vi "send_health_AURA.vi"(0 "TEMPERATURA":bool, 1 "Parametros AuraWheel":string[](array[string])=["nem1234", "test_rest", "http://api.aurawheel.dev/services/devices/status"], 2 "all rows":dbl[][](array[numeric]), 3 "WHEEL_SENSOR":bool, 4 "LIMITE MAX":dbl, 5 "LIMITE MIN":dbl, 6 "RFID_Error":errorcluster, 7 "FOTOCELULA":bool, 8 "RFID_LR6_Error":errorcluster, 9 "ESCRITURA ERROR":errorcluster, 10 "FPGA ERROR":errorcluster) -> (14 "JSON String Out":string, 15 "Response headers":string, 16 "error AURA":errorcluster)   [LabVIEW 2015]
uses:
  AURA_Wheel/Json2Labv.lvlib
panel:
  in  "DC":bool
  out "data":cluster{"status":string}
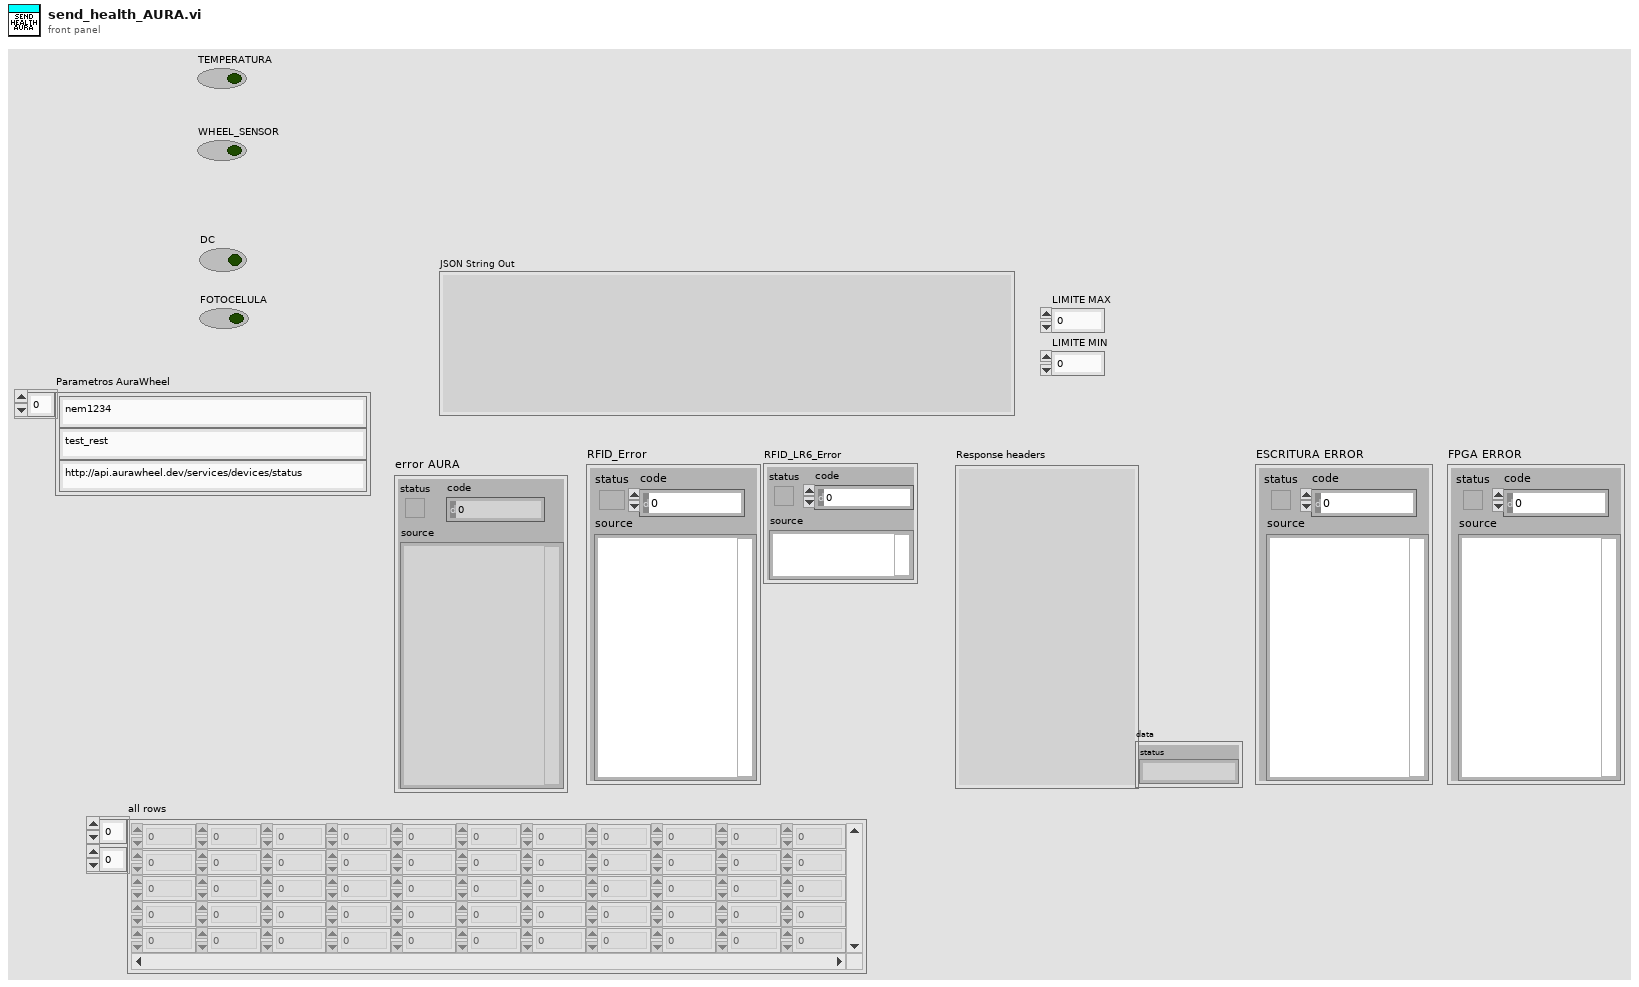
[diagram p1: front panel]
types:
  T1 = cluster{"g_st":dbl, "g_ts":dbl, "ds_id":string, "ds_st":dbl, "ds_ts":dbl, "ds_ss":cluster{"ss_tp":string, "ss_st":dbl, "ss_sl":string}[]}
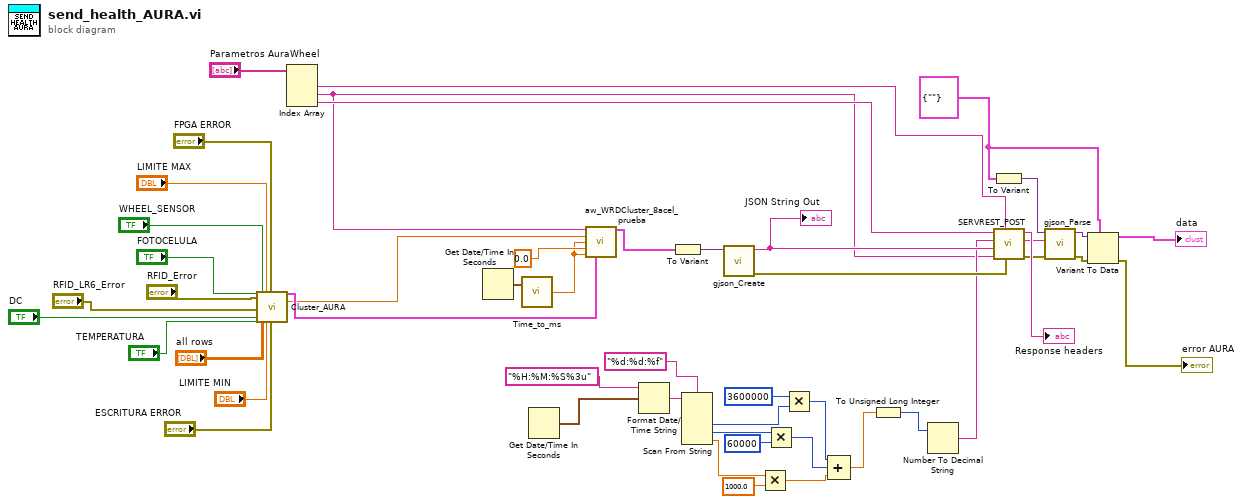
[diagram p0: block diagram]
diagram:
  w21 = cluster{"status":string} {"status"=""}
  n1 = call "Cluster_AURA.vi"("FOTOCELULA"="FOTOCELULA", "RFID_Error"="RFID_Error", "RFID_LR6_Error"="RFID_LR6_Error", "DC"="DC", "TEMPERATURA"="TEMPERATURA", "WHEEL_SENSOR"="WHEEL_SENSOR", "all rows"="all rows", "LIMITE MAX"="LIMITE MAX", "LIMITE MIN"="LIMITE MIN", "ERROR FPGA"="FPGA ERROR", "ERROR ESCRITURA"="ESCRITURA ERROR") -> ("appended array"=w45:cluster{string, dbl, "output string":string}[], "ESTADO WRD"=w11:dbl)  [unwired: 15 in]
  n2 = Index Array(array="Parametros AuraWheel") -> (element #1=w39:string, element #2=w4:string, element #3=w6:string)  [unwired: 3 in]
  n3 = Get Date/Time In Seconds() -> (seconds since 1Jan1904=w48:timestamp)
  n4 = call "Time_to_ms.vi"("seconds since 1Jan1904"=w48) -> ("Numeric"=w1:dbl)  [unwired: 1 in]
  n5 = Get Date/Time In Seconds() -> (seconds since 1Jan1904=w38:timestamp)
  n6 = call "aw_WRDCluster_8acel_prueba.vi"("ds_id"=w4, "ds_ss"=w45, "ds_st"=w11, "g_ts"=w1, "g_st"=0.0, "ds_ts"=w1) -> ("output cluster"=w47:T1)  [unwired: 9 in]
  n7 = Format Date/Time String(time format string (%c)="%H:%M:%S%3u", seconds (now)=w38) -> (date/time string=w36:string)  [unwired: 1 in]
  n8 = To Variant(anything=w47) -> (Variant=w49:variant)
  n9 = Scan From String(format string="%d:%d:%f", input string=w36) -> (output 1=w33:i32, output 2=w32:i32, output 3=w30:dbl)  [unwired: 5 in, 3 out]
  n10 = call "gjson_Create.vi"("JSON Object in"=w49) -> ("error out"=w16:errorcluster, "JSON String Out"=w7:string)  [unwired: 9 in]
  "JSON String Out" <- w7
  n11 = Multiply(x=w30, y=1000.0) -> (x*y=w26:dbl)
  n12 = Multiply(x=w32, y=60000) -> (x*y=w27:i32)
  n13 = Multiply(x=3600000, y=w33) -> (x*y=w28:i32)
  n14 = Compound Arithmetic op=ADD(w28, w27, w26) -> (w25:dbl)
  n15 = To Unsigned Long Integer(number=w25) -> (unsigned 32bit integer=w24:u32)
  n16 = Number To Decimal String(number=w24) -> (decimal integer string=w5:string)  [unwired: 1 in]
  n17 = To Variant(anything=w21) -> (Variant=w20:variant)
  n18 = call "SERVREST_POST.vi"("error in"=w16, "pwd"=w39, "User"=w4, "JSON Object"=w7, "x-nem-datetime"=w5, "URL"=w6) -> ("error out"=w22:errorcluster, "Response JSON"=w23:string, "Response headers"=→"Response headers":string)  [unwired: 3 in]
  n19 = call "gjson_Parse.vi"("error in"=w22, "JSON String In"=w23, "JSON Cluster"=w20) -> ("error out"=w18:errorcluster, "JSON Cluster Out"=w19:variant)  [unwired: 7 in]
  n20 = Variant To Data(error in=w18, type=w21, Variant=w19) -> (data=→"data":cluster{"status":string}, error out=→"error AURA":errorcluster)
